vi "swabian_disconnect.vi"(8 "error in (no error)":errorcluster, 11 "swabian_local_data_IN":T1={"events"={"update_status"=refnum, "update_chart"=refnum, "update_xy"=refnum, "send_channel_data"=refnum}, "stop_q"=refnum, "tagger_reference"=refnum, "connect_button"=refnum, "counter_reference"=refnum, "tagger_stream_reference"=refnum, "log_reference"=refnum, "current_log_offset"=0, "tt20_buffer_q"=refnum, "stream_to_file_button"=refnum, "num_records"=0, "connected?"=FALSE, "plots"=refnum, "histogram_bin_edges"=[], "histogrammer"=refnum, "plot_lifetimes"=refnum, "xy_graph"=refnum, "Reference\nChannel"=enum."ch0", "trigger_channels"=[], "filter_channels"=[], "active_channels"=[], "acq_mode"=0, "Reference\nChannel"=enum."ch0", "acq_time"=0, "sync_period_ps"=0, "raw_stream_path"=path "", "Leftovers"={"missing_sync_data"=[], "missing_events"=0}, "first_batch"=0, "first_sync_stamp"=0, "lifetime_settings"={"Plot Lifetimes"=FALSE, "start_time"=0.0, "stop_time"=0.0, "n_bins"=0}, "Histogram_bins"=[], "last_processed_data"=[], "histogram_data"=[]}) -> (0 "error out":errorcluster, 3 "swabian_local_data":T1={"events"={"update_status"=refnum, "update_chart"=refnum, "update_xy"=refnum, "send_channel_data"=refnum}, "stop_q"=refnum, "tagger_reference"=refnum, "connect_button"=refnum, "counter_reference"=refnum, "tagger_stream_reference"=refnum, "log_reference"=refnum, "current_log_offset"=0, "tt20_buffer_q"=refnum, "stream_to_file_button"=refnum, "num_records"=0, "connected?"=FALSE, "plots"=refnum, "histogram_bin_edges"=[], "histogrammer"=refnum, "plot_lifetimes"=refnum, "xy_graph"=refnum, "Reference\nChannel"=enum."ch0", "trigger_channels"=[], "filter_channels"=[], "active_channels"=[], "acq_mode"=0, "Reference\nChannel"=enum."ch0", "acq_time"=0, "sync_period_ps"=0, "raw_stream_path"=path "", "Leftovers"={"missing_sync_data"=[], "missing_events"=0}, "first_batch"=0, "first_sync_stamp"=0, "lifetime_settings"={"Plot Lifetimes"=FALSE, "start_time"=0.0, "stop_time"=0.0, "n_bins"=0}, "Histogram_bins"=[], "last_processed_data"=[], "histogram_data"=[]})   [LabVIEW 2018]
uses:
  swabian_local_data_tdef.ctl
  swabian_events_tdef.ctl
  update_chart_tdef.ctl
  channel_data_tdef.ctl
  C:/Users/bspoka/Documents/swabian_LV/lib/TTCSharp32.dll
  lib/TTCSharp32.dll
  swabian_buffer_tdef.ctl
  reference_checkbox_tdef.ctl
  lifetime_settings.ctl
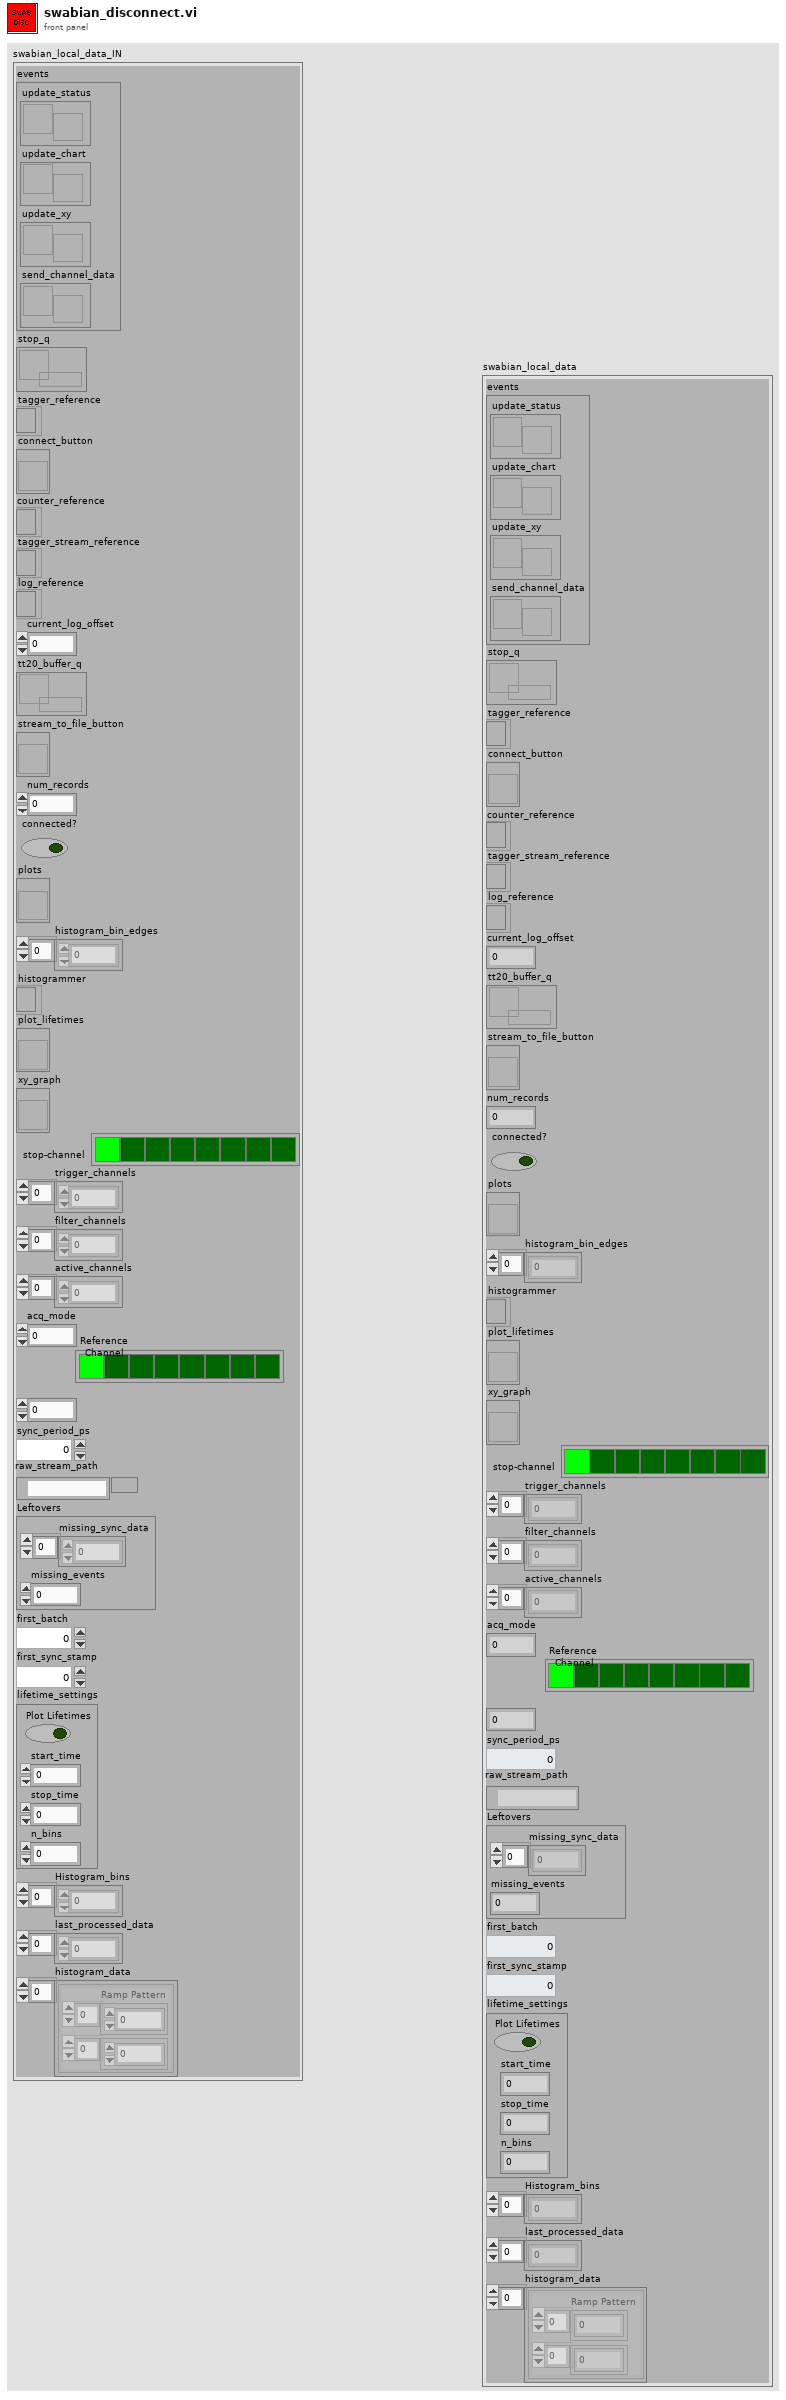
[diagram p1: front panel]
types:
  T1 = typedef "swabian_local_data_tdef.ctl" = cluster{"events":T2, "stop_q":refnum<queue>, "tagger_reference":refnum<k24>, "connect_button":refnum<vi>, "counter_reference":refnum<k24>, "tagger_stream_reference":refnum<k24>, "log_reference":refnum<file>, "current_log_offset":i64, "tt20_buffer_q":refnum<queue>, "stream_to_file_button":refnum<vi>, "num_records":u64, "connected?":bool, "plots":refnum<vi>, "histogram_bin_edges":i64[], "histogrammer":refnum<k24>, "plot_lifetimes":refnum<vi>, "xy_graph":refnum<vi>, "Reference\nChannel":T3, "trigger_channels":i32[], "filter_channels":i32[], "active_channels":i32[], "acq_mode":i32, "Reference\nChannel":T3, "acq_time":i64, "sync_period_ps":i64, "raw_stream_path":path, "Leftovers":cluster{"missing_sync_data":i64[], "missing_events":i32}, "first_batch":i32, "first_sync_stamp":i64, "lifetime_settings":T4, "Histogram_bins":dbl[], "last_processed_data":i64[], "histogram_data":cluster{"Ramp Pattern":dbl[], dbl[]}[]}
  T2 = typedef "swabian_events_tdef.ctl" = cluster{"update_status":refnum<user-event>, "update_chart":refnum<user-event>, "update_xy":refnum<user-event>, "send_channel_data":refnum<user-event>}
  T3 = typedef "reference_checkbox_tdef.ctl" = enum32{"No Selection", "ch0", "ch1", "ch2", "ch3", "ch4", "ch5", "ch6", "ch7"}
  T4 = typedef "lifetime_settings.ctl" = cluster{"Plot Lifetimes":bool, "start_time":dbl, "stop_time":dbl, "n_bins":i32}
  T5 = enum8{"Enabled", "Disabled", "Disabled and Grayed Out"}
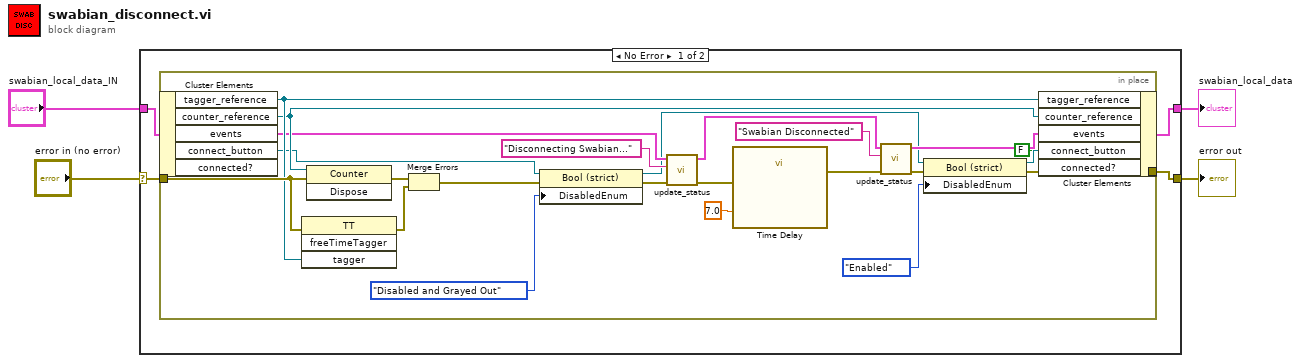
[diagram p0: block diagram]
diagram:
  n1 = case shown="No Error" "error in (no error)" {
    selector: "error in (no error)" -> [w7 w33]
    tunnel: "swabian_local_data_IN" -> [w8 w32]
    tunnel: [w6 w33] -> w2
    tunnel: [w5 w32] -> w1
    frame No Error {
      n2 = in-place {
        in-place-border: w7 -> [w28]
        in-place-border: [w10] -> w6
        n3 = in-place-cluster #1(w8) -> ("tagger_reference"=w27:refnum<k24>, "counter_reference"=w26:refnum<k24>, "events"=w23:T2, "connect_button"=w16:refnum<vi>)  [unwired: 1 out]
        n4 = invoke class="TT" method="freeTimeTagger"(error in=w28, "tagger"=w27) -> (error out=w29:errorcluster)  [unwired: 2 in, 3 out]
        n5 = invoke class="Counter" method="Dispose"(reference=w26, error in=w28) -> (error out=w30:errorcluster)  [unwired: 1 in, 2 out]
        n6 = Merge Errors(w30, w29) -> (w18:errorcluster)
        n7 = property class="Bool (strict)"(reference=w16, error in=w18, "DisabledEnum"=T5."Disabled and Grayed Out" ("Disabled")) -> (reference out=w13:refnum<vi>, error out=w17:errorcluster)
        n8 = call "update_status.vi"("error in (no error)"=w17, "status"="Disconnecting Swabian...", "events"=w23) -> ("error out"=w20:errorcluster, "events_out"=w22:T2)  [unwired: 7 in]
        n9 = call "Time Delay"("error in (no error)"=w20, "Delay Time (s)"=7.0) -> ("error out"=w19:errorcluster)  [unwired: 9 in]
        n10 = call "update_status.vi"("error in (no error)"=w19, "status"="Swabian Disconnected", "events"=w22) -> ("error out"=w11:errorcluster, "events_out"=w31:T2)  [unwired: 7 in]
        n11 = property class="Bool (strict)"(reference=w13, error in=w11, "DisabledEnum"=T5."Enabled" ("Disabled")) -> (reference out=w12:refnum<vi>, error out=w10:errorcluster)
        n12 = in-place-cluster #1("tagger_reference"=w27, "counter_reference"=w26, "events"=w31, "connect_button"=w12, "connected?"=FALSE) -> (w5:T1)
      }
    }
    frame Error {
    }
  }
  "error out" <- w2
  "swabian_local_data" <- w1
